vi "Initialise Variable length FIFO.vi"() -> (11 "FPGA VI Reference":T1)   [LabVIEW 2020]
uses:
  <vilib>/rvi/interface/nirviMethod/nirviMethod.xnode
  RIG-SPECIFIC FILES/FPGA Refs/FPGA Ref.ctl
  <vilib>/FPGAPlugInAG/Dynamic/niLvFpga_ConfigureFifo_Dynamic.vi
  <vilib>/rvi/errors/niLvFpgaMergeErrorWithErrorCode.vi
panel:
  in  "FPGA VI Reference":T1
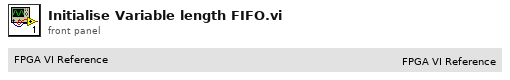
[diagram p1: front panel]
types:
  T1 = typedef "FPGA Ref.ctl" = refnum<k20>
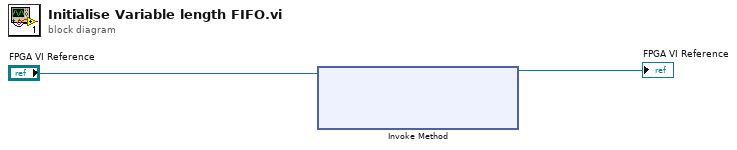
[diagram p0: block diagram]
diagram:
  n1 = xnode "Invoke Method"("FPGA VI Reference In"="FPGA VI Reference") -> ("FPGA VI Reference Out"=→"FPGA VI Reference":T1)  [unwired: 2 in, 2 out]
